vi "Obtain parse data changes event.vi"(8 "error in (no error)":errorcluster, 11 "Fiber Auto Collimation panel":refnum<class "Fiber Auto Collimation panel.lvclass">) -> (0 "error out":errorcluster, 3 "Parse data changes":refnum<user-event>)   [LabVIEW 2018, in "Fiber Auto Collimation References.lvclass"]
doc: "This VI gets the reference to an event that should be used only in a view loop to send a signal to itself containing an array of all of the state data contents that have just been updated.\n\nThis VI is set to use an array of raw U16 numbers and not the type definition for the state data tracking enum. It could be changed, but the event template copying does not handle it well so it was not set up that way in the template to avoid too many conflicts to resolve.\n\nBecause this event is created once per panel and once per clone, it should be destroyed right before the panel finally closes to avoid memory leaks."
uses:
  Fiber Auto Collimation References.lvclass
  Panels/Fiber Auto Collimation panel.lvclass
  C:/Program Files (x86)/National Instruments/LabVIEW 2018/user.lib/nLight Tidbits/Cross-library references/Cross-library key/Cross-library key.lvclass
  b47026bc-8271-46ff-bcce-21c2580a6587.vi
  f406f5ab-9891-41e2-b0a1-c13e850666b3.vi
  b47026bc-8271-46ff-bcce-21c2580a6587.vi/80a55534-07b4-46f3-95dc-9cfd723c105d.vi
  <userlib>/nLight Tidbits/Cross-library references/Cross-library key/Obtain cross library semaphore and acquire.vi
  b47026bc-8271-46ff-bcce-21c2580a6587.vi/4da48868-7ba5-4708-8795-12157d94ca14.vi
  f406f5ab-9891-41e2-b0a1-c13e850666b3.vi/53d4c5d6-f8c1-450b-89f8-0892ad8fc76d.vi
  f406f5ab-9891-41e2-b0a1-c13e850666b3.vi/861b9ba3-e80f-41d3-82b8-501c193dd8d2.vi
  <userlib>/nLight Error Handling/Trash error.vi
  <vilib>/Utility/error.llb/Clear Errors.vi
  <vilib>/Utility/semaphor.llb/Obtain Semaphore Reference.vi
  <vilib>/Utility/semaphor.llb/Acquire Semaphore.vi
  <userlib>/nLight Error Handling/Log any errors.vi
  <userlib>/nLight Tidbits/Cross-library references/Cross-library key/Obtain class key.vi
  <vilib>/Utility/semaphor.llb/Release Semaphore.vi
  <vilib>/Utility/semaphor.llb/Release Semaphore Reference.vi
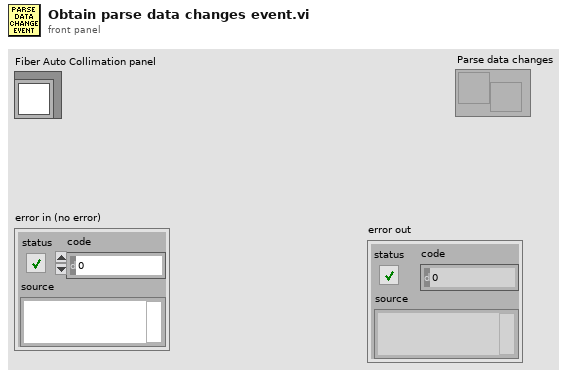
[diagram p1: front panel]
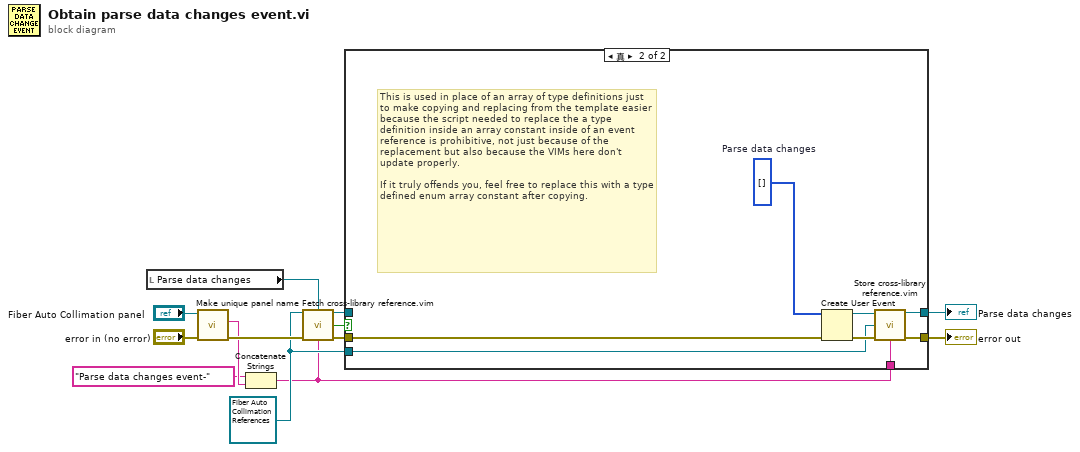
[diagram p0: block diagram]
diagram:
  w9 = refnum<class "Fiber Auto Collimation References.lvclass"> refnum ("nLight Station Template References.lvclass")
  n1 = local read "Parse data changes"() -> (w2:refnum<user-event>)
  n2 = call "Make unique panel name.vi"("error in (no error)"="error in (no error)", "Fiber Auto Collimation panel in"="Fiber Auto Collimation panel") -> ("error out"=w10:errorcluster, "Unique panel name"=w6:string)  [unwired: 7 in, 1 out]
  n3 = Concatenate Strings("Parse data changes event-" ("string"), w6) -> (w5:string)
  n4 = call "Fetch cross-library reference.vim"("Cross-library key"=w9, "Reference type to fetch"=w2, "error in (no error)"=w10, "Specific ref type name [String/Enum]"=w5) -> ("Stored value (if present)"=w1:refnum<user-event>, "Nothing to fetch OR bad reference"=w8:bool, "error out"=w7:errorcluster)  [unwired: 9 in]
  n5 = case shown="真" w8 {
    tunnel: w7 -> [w15 w23]
    tunnel: [w15 w20] -> w13
    tunnel: w9 -> [_ w19]
    tunnel: w5 -> [_ w18]
    tunnel: [w14 w17] -> w3
    tunnel: w1 -> [w14 _]
    frame False {
    }
    frame True {
      w16 = u16[] []  # Parse data changes
      # "This is used in place of an array of type definitions just to make copying and replacing from the template easier because the script needed to replace the a type definition inside an array constant inside of an event reference is prohibitive, not just because of the replacement but also because the VIMs here don't update properly.\n\nIf it truly offends you, feel free to replace this with a type defined enum array constant after copying."
      n6 = Create User Event(user event datatype=w16, error in=w23) -> (user event=w21:refnum<user-event>, error out=w22:errorcluster)
      n7 = call "Store cross-library reference.vim"("Reference to store"=w21, "Cross-library key"=w19, "error in (no error)"=w22, "Specific ref type name [String/Enum]"=w18) -> ("Copy of stored reference"=w17:refnum<user-event>, "error out"=w20:errorcluster)  [unwired: 8 in, 2 out]
    }
  }
  "error out" <- w13
  "Parse data changes" <- w3
